vi "SigMath_Create.vi"(0 "reference in":refnum<class "SigMath.lvclass">, 5 "error in (no error)":errorcluster, 6 "Time Data":refnum<class "GSwFormDSP.lvclass">, 7 "Application Name":string, 9 "State Queue":string[](array[string])) -> (14 "reference out":refnum<class "SigMath.lvclass">, 19 "error out":errorcluster)   [LabVIEW 2020, in "SigMath.lvclass"]
doc: "Constructor."
uses:
  SigMath.lvclass
  C:/Program Files/National Instruments/LabVIEW 2020/vi.lib/addons/_AddQ/G#Object/G#Object.lvclass
  C:/Users/fcharett/docsWork/coding/20SPWB/C/Users/fcharett/docsWork/coding/LabVIEW/API/Generic Utilities_class/Generic Utilities.lvclass
  API/GSwFormDSP_class/GSwFormDSP.lvclass
  <vilib>/addons/_AddQ/G#Object/G#Object.lvclass
  API/Generic Utilities_class/Generic Utilities.lvclass
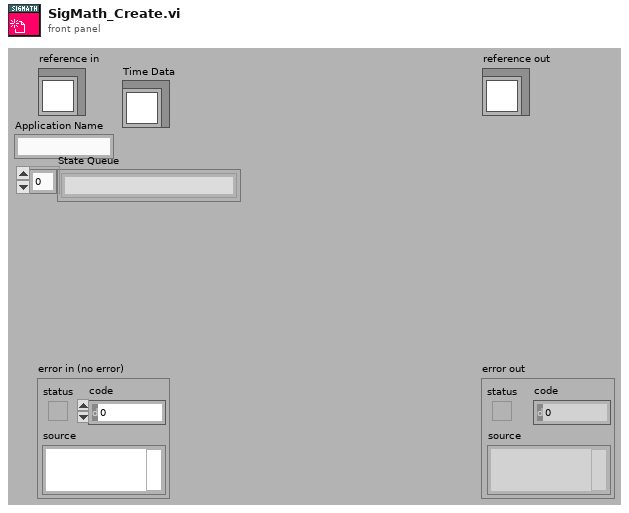
[diagram p1: front panel]
types:
  T1 = typedef "SigMath.lvclass/ObjectAttributesRef.ctl" = refnum<data-value>
  T2 = typedef "SigMath.lvclass/ObjectAttributes.ctl" = cluster{"SigMath Data":T3, "User CTRL Refs":T4}
  T3 = typedef "SigMath.lvclass/SigMath Data.ctl" = cluster{"New Time Data Obj?":bool, "GSwFormDSP":refnum<class "GSwFormDSP.lvclass">}
  T4 = typedef "SigMath.lvclass/SigMath User CTRL Refs.ctl" = cluster{"wForms":refnum<vi>, "Results wForms":refnum<vi>}
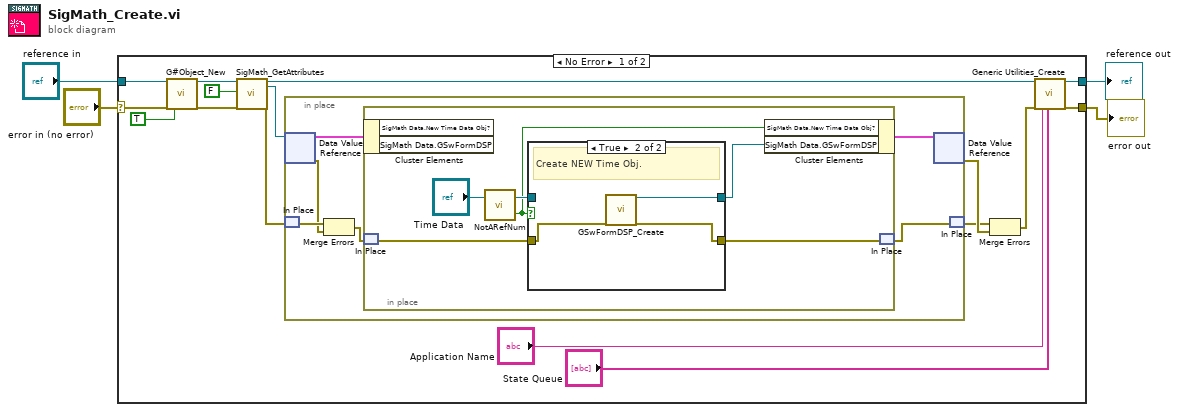
[diagram p0: block diagram]
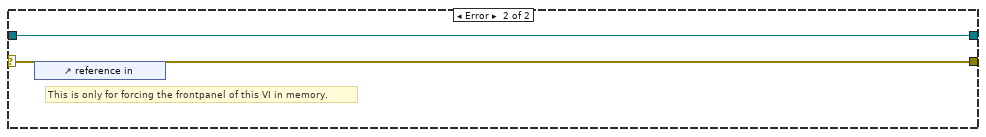
[diagram p3: hidden frame]
diagram:
  n1 = case shown="No Error" "error in (no error)" {
    selector: "error in (no error)" -> [w19 w39]
    tunnel: [w10 w39] -> w3
    tunnel: [w12 w38] -> w1
    tunnel: "reference in" -> [w20 w38]
    frame No Error {
      n2 = call <vilib>:"G#Object_New.vi"("reference in"=w20, "error in (no error)"=w19, "user counter (T)?"=TRUE ("User Counter")) -> ("reference out"=w15:refnum<class "SigMath.lvclass">, "error out"=w14:errorcluster)  [unwired: 14 in, 1 out]
      n3 = call "SigMath_GetAttributes.vi"("reference in"=w15, "return data? (T)"=FALSE ("return data"), "error in (no error)"=w14) -> ("reference out"=w13:refnum<class "SigMath.lvclass">, "attributes ref"=w8:T1, "error out"=w7:errorcluster)  [unwired: 13 in, 1 out]
      n4 = in-place {
        n5 = in-place-dvr #1(w8) -> (w25:T2, w23:errorcluster)
        n6 = in-place-match #2(w7) -> (w24:errorcluster)
        n7 = Merge Errors(w24, w23) -> (w22:errorcluster)
        n8 = in-place {
          n9 = in-place-cluster #3(w25) -> ()  [unwired: 2 out]
          n10 = in-place-match #4(w22) -> (w30:errorcluster)
          n11 = call-dynamic "NotARefNum.vi"("reference in"="Time Data") -> ("not a refnum?"=w27:bool, "reference out"=w31:refnum<class "GSwFormDSP.lvclass">)  [unwired: 1 in]
          n12 = case shown="True" w27 {
            tunnel: [w34 w35] -> w29
            tunnel: w31 -> [w34 _]
            tunnel: w30 -> [w33 w37]
            tunnel: [w33 w36] -> w28
            frame False {
              # "Copy an existing reference."
            }
            frame True {
              # "Create NEW Time Obj."
              n13 = call "GSwFormDSP_Create.vi"("error in (no error)"=w37) -> ("reference out"=w35:refnum<class "GSwFormDSP.lvclass">, "error out"=w36:errorcluster)  [unwired: 17 in]
            }
          }
          n14 = in-place-cluster #3("SigMath Data.New Time Data Obj?"=w27, "SigMath Data.GSwFormDSP"=w29) -> (w26:T2)
          n15 = in-place-match #4(w28) -> (w21:errorcluster)
        }
        n16 = in-place-dvr #1(w26) -> (w17:errorcluster)  [unwired: 1 out]
        n17 = in-place-match #2(w21) -> (w6:errorcluster)
      }
      n18 = Merge Errors(w6, w17) -> (w11:errorcluster)
      n19 = call "Generic Utilities_Create.vi"("reference in"=w13, "error in (no error)"=w11, "Application Name"="Application Name", "State Queue"="State Queue") -> ("reference out"=w12:refnum<class "SigMath.lvclass">, "error out"=w10:errorcluster)  [unwired: 14 in]
    }
    frame Error {
      # "This is only for forcing the frontpanel of this VI in memory."
      n20 = control-ref of="reference in"() -> ()  [unwired: 1 out]
    }
  }
  "error out" <- w3
  "reference out" <- w1
